vi "set_objectName.vi"(0 "HGF_Factory":refnum<class "HGF_Factory.lvclass">, 2 "objectName":string, 5 "error in (no error)":errorcluster) -> (14 "dup HGF_Factory":refnum<class "HGF_Factory.lvclass">, 19 "error out":errorcluster)   [LabVIEW 2014, in "HGF_BaseClasses.lvlib" / "HGF_Factory.lvclass"]
doc: "Set name of object."
uses:
  HGF_Factory.lvclass
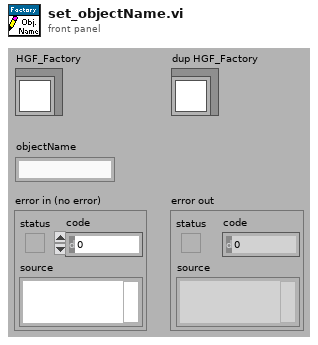
[diagram p1: front panel]
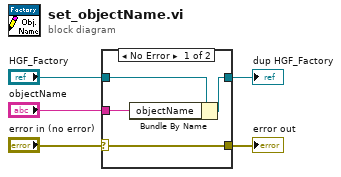
[diagram p0: block diagram]
diagram:
  n1 = case shown="No Error" "error in (no error)" {
    selector: "error in (no error)" -> [w9 w10]
    tunnel: [w9 w10] -> w4
    tunnel: [w7 w11] -> w2
    tunnel: "HGF_Factory" -> [w8 w11]
    tunnel: "objectName" -> [w6 _]
    frame No Error {
      n2 = Bundle By Name(cluster=w8, "objectName"=w6) -> (w7:refnum<class "HGF_Factory.lvclass">)
    }
    frame Error {
    }
  }
  "error out" <- w4
  "dup HGF_Factory" <- w2
